vi "Update Watchdog Status.vi"(8 "Error In":errorcluster, 10 "Watchdog Status":T1, 11 "CS++RTMainActor in":refnum<class "CS++RTMainActor.lvclass">) -> (0 "Error Out":errorcluster, 3 "CS++RTMainActor out":refnum<class "CS++RTMainActor.lvclass">)   [LabVIEW 2016, in "CS++RTMain.lvlib" / "CS++RTMainActor.lvclass"]
doc: "Update watchdog status. This VI stores the new status in its own attribute and calls the corresponding dynamic dispatch core implementation."
uses:
  CS++RTMain/CS++RTMainActor.lvclass
  <vilib>/RTwatchdog.llb/Watchdog status enum.ctl
  CS++RTMain/CS++RTMainActor.lvclass/CS++RTMainActor.ctl
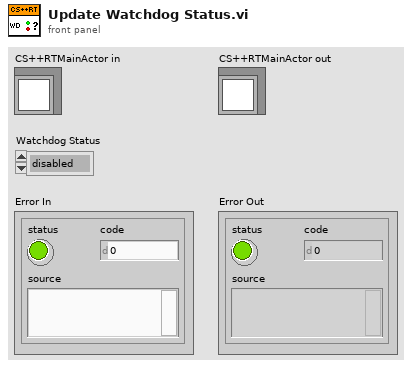
[diagram p1: front panel]
types:
  T1 = typedef "Watchdog status enum.ctl" = enum16{"disabled", "expired", "running"}
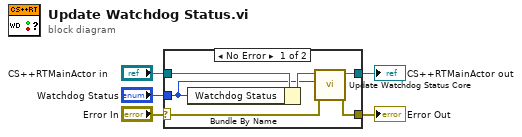
[diagram p0: block diagram]
diagram:
  n1 = case shown="No Error" "Error In" {
    selector: "Error In" -> [w6 w13]
    tunnel: [w7 w13] -> w4
    tunnel: [w8 w12] -> w1
    tunnel: "CS++RTMainActor in" -> [w11 w12]
    tunnel: "Watchdog Status" -> [w9 _]
    frame No Error {
      n2 = Bundle By Name(cluster=w11, "Watchdog Status"=w9) -> (w10:refnum<class "CS++RTMainActor.lvclass">)
      n3 = call-dynamic "Update Watchdog Status Core.vi"("Error In"=w6, "watchdog status"=w9, "CS++RTMainActor in"=w10) -> ("Error Out"=w7:errorcluster, "CS++RTMainActor out"=w8:refnum<class "CS++RTMainActor.lvclass">)  [unwired: 7 in]
    }
    frame Error {
    }
  }
  "Error Out" <- w4
  "CS++RTMainActor out" <- w1
